vi "Start Master.vi"(8 "error in (no error)":errorcluster, 11 "Kasli Wrapper in":refnum<class "Kasli Wrapper 2.0.lvclass">) -> (0 "error out":errorcluster, 3 "Kasli Wrapper out":refnum<class "Kasli Wrapper 2.0.lvclass">)   [LabVIEW 2020, in "TALOS.lvlib" / "Kasli Wrapper 2.0.lvlib" / "Kasli Wrapper 2.0.lvclass"]
uses:
  Kasli Wrapper 2.0.lvclass
  Kasli Wrapper 2.0.lvclass/Kasli Wrapper 2.0.ctl
  Ancestor/Ancestor/Ancestor.lvclass/Ancestor.ctl
  Support VIs/Generate Error.vi
  FGV/Error Memory/Get Error Description.vi
  Support VIs/Get PC name.vi
  Ancestor/Ancestor/Read ID.vi
  Support VIs/Get Class Name.vi
  <vilib>/Utility/error.llb/Clear Errors.vi
  FGV/Error Memory/Error Memory Core.vi
  <vilib>/AdvancedString/Delimited String to 1D String Array.vi
  Support VIs/Circus Root Path.vi
  FGV/Error Memory/Error Crt Lvl checker.vi
  FGV/Error Memory/Error Memory Core.vi/40c8088d-b597-4017-91af-faa98e00292e.vi
  FGV/Error Memory/Error Memory Core.vi/d4a3ab98-063c-4e44-b43d-fbdcfe6c2be2.vi
  <vilib>/Utility/error.llb/Search and Replace Pattern.vi
  Support VIs/Global Memory.vi
  <vilib>/Utility/LVClass/Get LV Class Name.vi
  Support VIs/Is in Packed Library.vi
  Support VIs/TALOS Root path.vi
  Support VIs/Read CSV worksheet.vi
  Support VIs/Global Constants.vi
  <vilib>/Utility/error.llb/General Error Handler.vi
  Support VIs/Error Log.vi
  Ancestor/Ancestor/Ancestor.lvclass
  <vilib>/Comparison/Equal/Equal Functor/Equal Functor.lvclass
  Kasli/Kasli.lvclass
  builds/JKI dotNET System Exec/JKI_dotNET_System_Exec_PPL.lvlibp/dotnet_system_exec.lvclass
  TALOS.lvlib
  Kasli Wrapper 2.0.lvlib
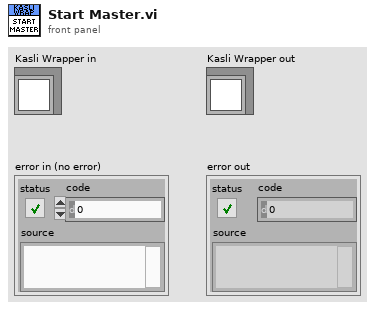
[diagram p1: front panel]
types:
  T1 = cluster{"stdout event":refnum<user-event>, "stderr event":refnum<user-event>, "process_exit event":refnum<user-event>}
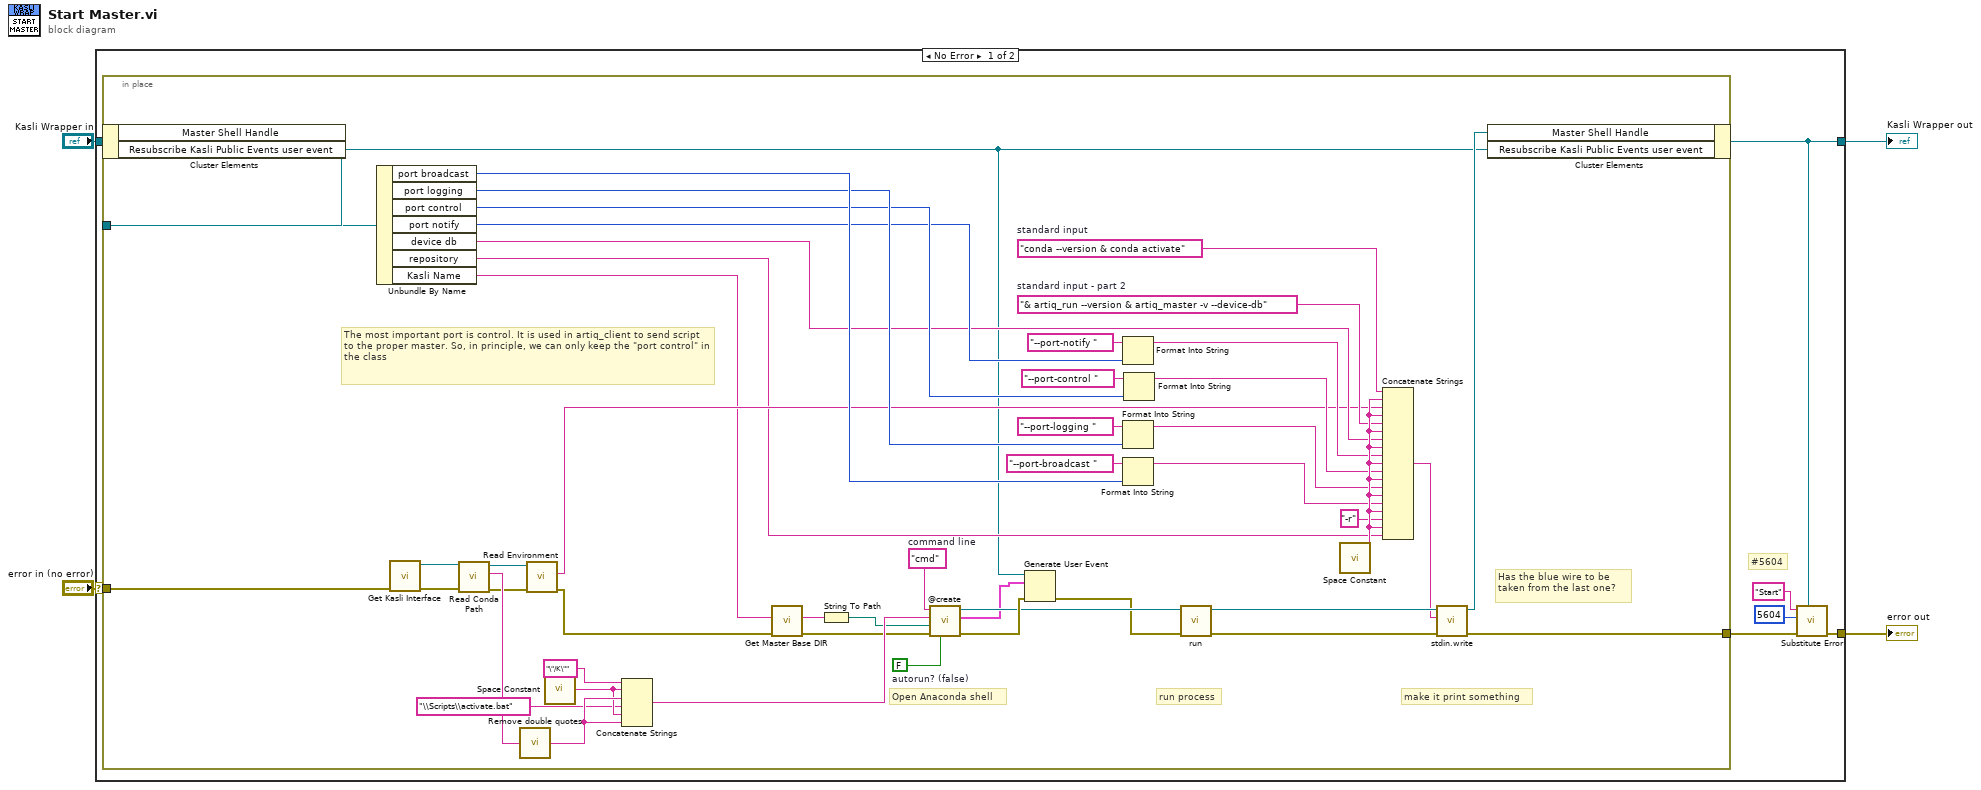
[diagram p0: block diagram]
diagram:
  n1 = case shown="No Error" "error in (no error)" {
    selector: "error in (no error)" -> [w11 w60]
    tunnel: [w6 w61] -> w4
    tunnel: [w7 w60] -> w3
    tunnel: "Kasli Wrapper in" -> [w10 w61]
    frame No Error {
      # "#5604"
      n2 = in-place {
        in-place-border: w11 -> [w53]
        in-place-border: [w23] -> w8
        in-place-border: w10 -> [w42]
        w44 = "& artiq_run --version & artiq_master -v --device-db"  # standard input - part 2
        w43 = "conda --version & conda activate"  # standard input
        w29 = FALSE  # autorun? (false)
        w34 = "cmd"  # command line
        # "The most important port is control. It is used in artiq_client to send script to the proper master. So, in principle, we can only keep the \"port control\" in the class"
        # "make it print something"
        # "Has the blue wire to be taken from the last one?"
        # "run process"
        # "Open Anaconda shell"
        n3 = in-place-cluster #1(w10) -> ("Resubscribe Kasli Public Events user event"=w13:refnum<user-event>)  [unwired: 1 out]
        n4 = Unbundle By Name(w42) -> ("port broadcast"=w41:u32, "port logging"=w40:u32, "port control"=w39:u32, "port notify"=w38:u32, "device db"=w37:string, "repository"=w20:string, "Kasli Name"=w19:string)
        n5 = call "Get Kasli Interface.vi"("error in"=w53) -> ("error out"=w16:errorcluster, "Kasli Interface"=w17:refnum<class "Kasli.lvclass">)  [unwired: 9 in]
        n6 = call-dynamic "Read Conda Path.vi"("error in (no error)"=w16, "Kasli in"=w17) -> ("error out"=w18:errorcluster, "Conda Path"=w57:string, "Kasli out"=w15:refnum<class "Kasli.lvclass">)  [unwired: 7 in]
        n7 = call "Remove double quotes.vi"("Input string"=w57) -> ("Output string"=w58:string)  [unwired: 4 in]
        n8 = call-dynamic "Read Environment.vi"("error in (no error)"=w18, "Kasli in"=w15) -> ("error out"=w36:errorcluster, "Environment"=w21:string)  [unwired: 7 in, 1 out]
        n9 = call <vilib>:"Space Constant.vi"() -> ("String"=w56:string)
        n10 = Concatenate Strings("\"/K\"", w56, w58, "\\Scripts\\activate.bat" ("string"), w56, w58) -> (w33:string)
        n11 = call "Get Master Base DIR.vi"("error in (no error)"=w36, "relative path"=w19) -> ("error out"=w31:errorcluster, "Master DIR"=w14:string)  [unwired: 4 in]
        n12 = String To Path(string=w14) -> (path=w32:path)
        n13 = call "@create.vi"("autorun? (false)"=w29, "error in (no error)"=w31, "working directory (c:\\)"=w32, "arguments (\"\")"=w33, "command line (cmd.exe)"=w34) -> ("error out"=w30:errorcluster, "public events"=w12:T1, "dotnet_system_exec out"=w28:refnum<class "dotnet_system_exec.lvclass">)  [unwired: 4 in]
        n14 = Generate User Event(user event=w13, event data cluster=w12, error in=w30) -> (error out=w27:errorcluster)  [unwired: 1 in, 1 out]
        n15 = Format Into String(initial string="--port-notify ", w38) -> (resulting string=w48:string)  [unwired: 2 in, 1 out]
        n16 = Format Into String(initial string="--port-logging ", w40) -> (resulting string=w46:string)  [unwired: 2 in, 1 out]
        n17 = Format Into String(initial string="--port-broadcast ", w41) -> (resulting string=w45:string)  [unwired: 2 in, 1 out]
        n18 = Format Into String(initial string="--port-control ", w39) -> (resulting string=w47:string)  [unwired: 2 in, 1 out]
        n19 = call "run.vi"("error in (no error)"=w27, "dotnet_system_exec in"=w28) -> ("error out"=w24:errorcluster, "dotnet_system_exec out"=w26:refnum<class "dotnet_system_exec.lvclass">)  [unwired: 8 in]
        n20 = call <vilib>:"Space Constant.vi"() -> ("String"=w59:string)
        n21 = Concatenate Strings(w43, w59, w21, w59, w44, w59, w37, w59, w48, w59, w47, w59, w46, w59, w45, w59, "-r" ("string"), w59, w20) -> (w25:string)
        n22 = call-dynamic "stdin.write.vi"("error in (no error)"=w24, "stdin"=w25, "dotnet_system_exec in"=w26) -> ("error out"=w23:errorcluster, "dotnet_system_exec out"=w22:refnum<class "dotnet_system_exec.lvclass">)  [unwired: 7 in]
        n23 = in-place-cluster #1("Master Shell Handle"=w22, "Resubscribe Kasli Public Events user event"=w13) -> (w6:refnum<class "Kasli Wrapper 2.0.lvclass">)
      }
      n24 = call "Substitute Error.vi"("LabVIEW Object"=w6, "error in (no error)"=w8, "Error Code"=5604, "Optional String"="Start") -> ("error out"=w7:errorcluster)  [unwired: 7 in]
    }
    frame Error {
    }
  }
  "Kasli Wrapper out" <- w4
  "error out" <- w3
